vi "Initial Setup.vi"(8 "Team Index":i32, 9 "Column":i32, 10 "Row":i32, 11 "Runner":refnum<class "AntFarm_MB.lvclass">) -> (1 "Column Out":i32, 2 "Row Out":i32, 3 "Runner Out":refnum<class "AntFarm_MB.lvclass">)   [LabVIEW 2016, in "AntFarm_MB.lvclass"]
uses:
  AntFarm_MB.lvclass
  TypeDefs/Cluster_Ant Farm Global Data.ctl
  AntFarm_MB.lvclass/AntFarm_MB.ctl
  SubVIs/Read-Only Globals.vi
  SubVIs/Globals (private).vi
  Square/Square.lvclass
panel:
  out "Global Data":T1
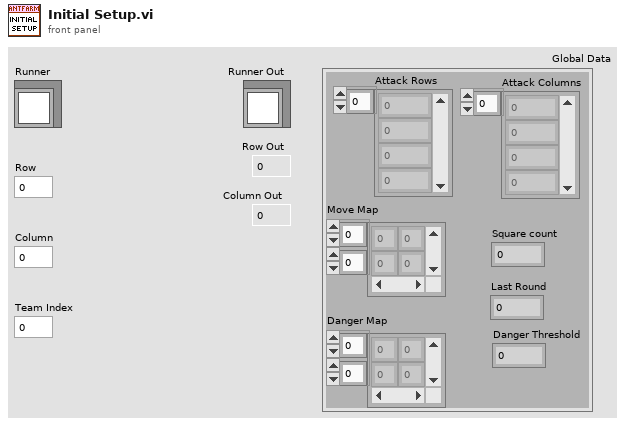
[diagram p1: front panel]
types:
  T1 = typedef "Cluster_Ant Farm Global Data.ctl" = cluster{"Move Map":i32[][], "Danger Map":i32[][], "Attack Rows":i32[], "Attack Columns":i32[], "Square count":i32, "Last Round":i32, "Danger Threshold":i32}
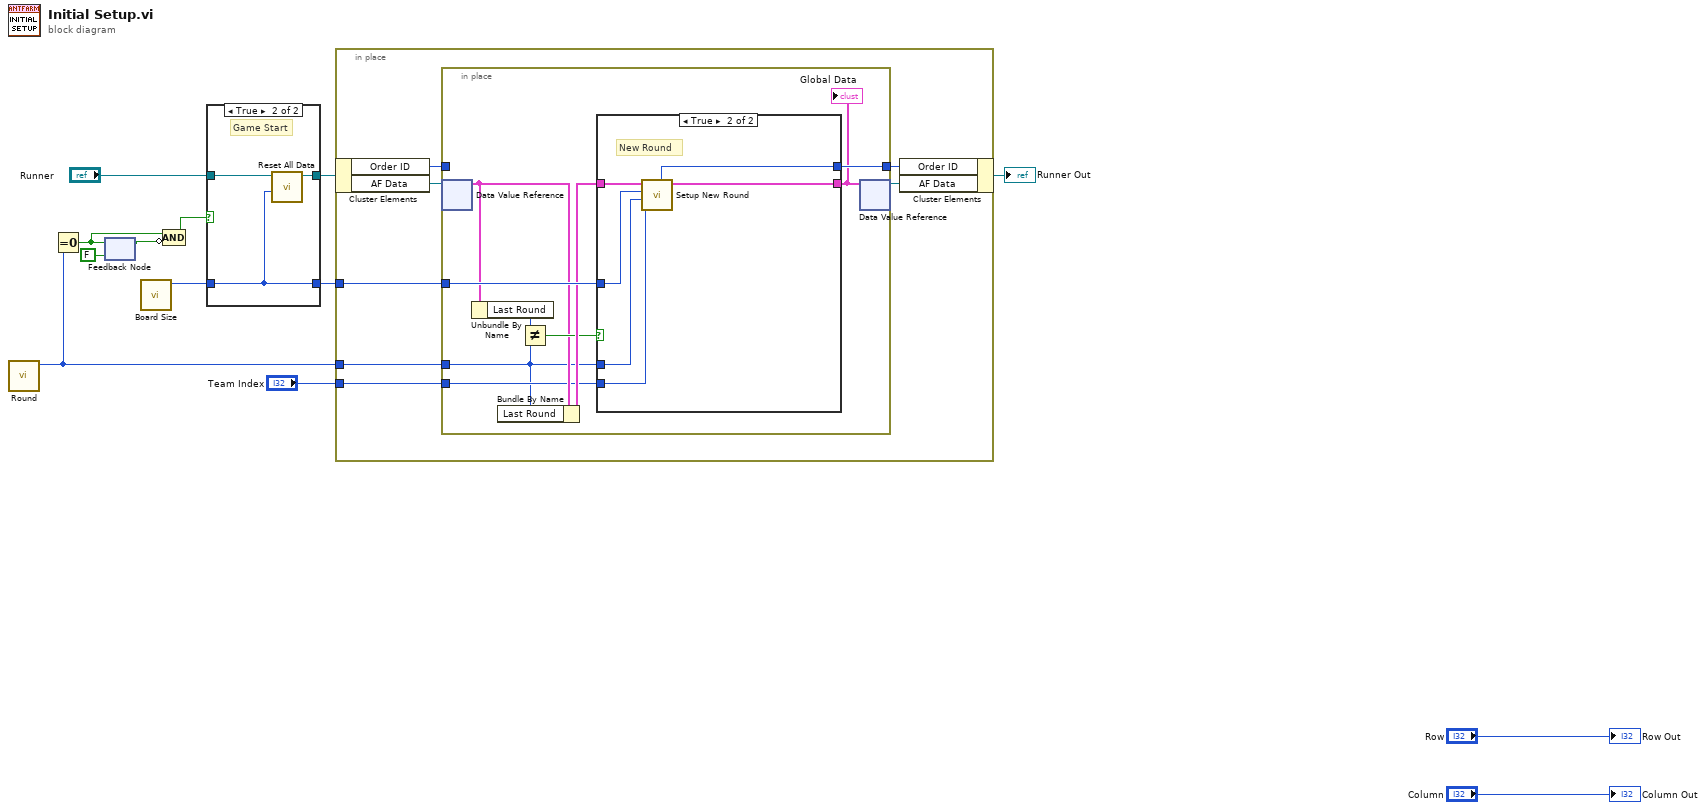
[diagram p0: block diagram]
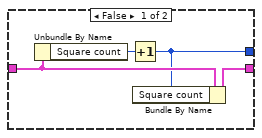
[diagram p2: hidden frame]
diagram:
  n1 = call "Round.vi"() -> ("Round"=w10:i32)  [unwired: 11 in]
  n2 = Equal To 0?(x=w10) -> (x = 0?=w7:bool)
  n3 = feedback #1(FALSE) -> (w8:bool)
  n4 = feedback-in #1(w7) -> ()
  n5 = call "Board Size.vi"() -> ("Board Size"=w11:i32)  [unwired: 11 in]
  n6 = Compound Arithmetic op=AND(w7, invert w8) -> (w6:bool)
  n7 = case shown="True" w6 {
    tunnel: [w15 w18] -> w13
    tunnel: "Runner" -> [w14 w17]
    tunnel: [w14 w16] -> w3
    tunnel: w11 -> [w15 w18]
    frame False {
    }
    frame True {
      # "Game Start"
      n8 = call "Reset All Data.vi"("Board Size"=w18, "AntFarm_MB"=w17) -> ("AntFarm_MB Out"=w16:refnum<class "AntFarm_MB.lvclass">)  [unwired: 9 in]
    }
  }
  n9 = in-place {
    in-place-border: w13 -> [w25]
    in-place-border: w10 -> [w24]
    in-place-border: "Team Index" -> [w19]
    n10 = in-place-cluster #2(w3) -> ("Order ID"=w21:i32, "AF Data"=w23:refnum<data-value>)
    n11 = in-place {
      in-place-border: w25 -> [w34]
      in-place-border: [w33] -> w20
      in-place-border: w24 -> [w26]
      in-place-border: w21 -> [_]
      in-place-border: w19 -> [w27]
      n12 = in-place-dvr #3(w23) -> (w28:T1)  [unwired: 1 out]
      n13 = Unbundle By Name(w28) -> ("Last Round"=w30:i32)
      n14 = Bundle By Name(cluster=w28, "Last Round"=w26) -> (w32:T1)
      n15 = Not Equal?(x=w30, y=w26) -> (x != y?=w31:bool)
      n16 = case shown="True" w31 {
        tunnel: w34 -> [_ w41]
        tunnel: w32 -> [w37 w44]
        tunnel: [w36 w43] -> w29
        tunnel: [w35 w42] -> w33
        tunnel: w27 -> [_ w40]
        tunnel: w26 -> [_ w39]
        frame False {
          n17 = Unbundle By Name(w37) -> ("Square count"=w38:i32)
          n18 = Increment(x=w38) -> (x+1=w35:i32)
          n19 = Bundle By Name(cluster=w37, "Square count"=w35) -> (w36:T1)
        }
        frame True {
          # "New Round"
          n20 = call "Setup New Round.vi"("Team Index"=w40, "Round"=w39, "Board Size"=w41, "Global Data"=w44) -> ("Global Data Out"=w43:T1, "Data.Order ID Out"=w42:i32)  [unwired: 6 in]
        }
      }
      "Global Data" <- w29
      n21 = in-place-dvr #3(w29) -> (w22:refnum<data-value>)  [unwired: 1 out]
    }
    n22 = in-place-cluster #2("Order ID"=w20, "AF Data"=w22) -> (→"Runner Out":refnum<class "AntFarm_MB.lvclass">)
  }
  "Row Out" <- "Row"
  "Column Out" <- "Column"
